vi "GetClassImplementationTypeDefNames.vi"(8 "error in (no error)":errorcluster, 11 "ClassReaderNative in":refnum<class "ClassReaderNative.lvclass">) -> (0 "error out":errorcluster, 2 "ImplementationMethodNames":string[](array[string]), 3 "ClassReaderNative out":refnum<class "ClassReaderNative.lvclass">)   [LabVIEW 2016, in "ClassReaderNative.lvclass"]
uses:
  <resource>/Framework/Providers/Open_GDS/ClassProviders/Provider_LvNativeClass/ClassReaderNative_class/ClassReaderNative.lvclass
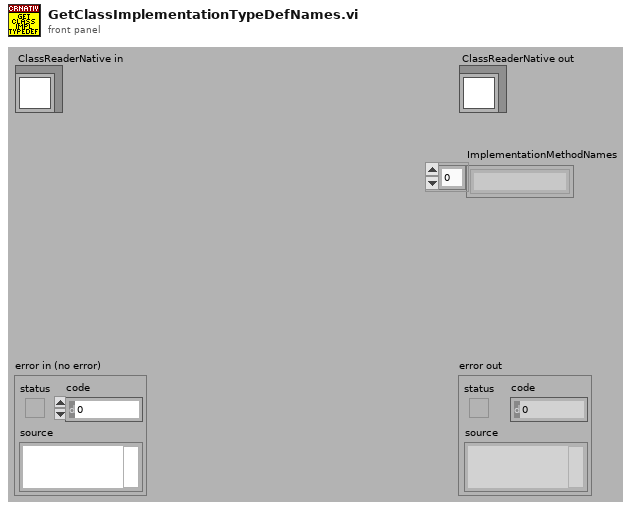
[diagram p1: front panel]
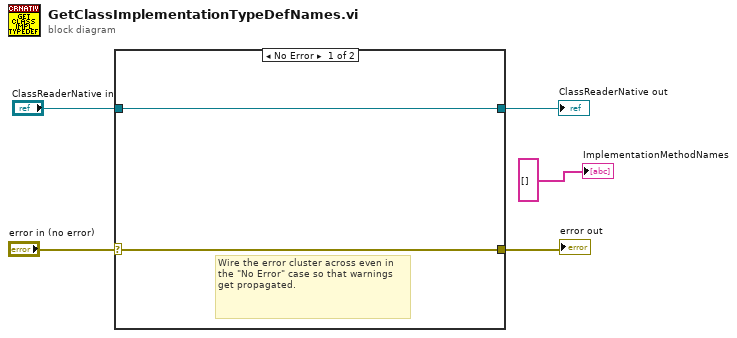
[diagram p0: block diagram]
diagram:
  n1 = case shown="No Error" "error in (no error)" {
    selector: "error in (no error)" -> [w6 w9]
    tunnel: [w6 w9] -> w4
    tunnel: [w7 w8] -> w2
    tunnel: "ClassReaderNative in" -> [w7 w8]
    frame No Error {
      # "Wire the error cluster across even in the \"No Error\" case so that warnings get propagated."
    }
    frame Error {
    }
  }
  "error out" <- w4
  "ClassReaderNative out" <- w2
  "ImplementationMethodNames" <- string[] [] ("ImplementationMethodNames")
